vi "CAN BL Node Check.vi"(5 "TimeOut":u32, 6 "pType":u32, 7 "pVersion":u32, 9 "NodeAddr":u16, 10 "CANIndex":i32, 11 "DevHandle":i32) -> (2 "function return":i32, 3 "pVersion out":u32, 4 "pType out":u32)   [LabVIEW 2010, in "usb2can.lvlib"]
doc: "int WINAPI CAN_BL_NodeCheck(int DevHandle,int CANIndex,unsigned short NodeAddr,unsigned int *pVersion,unsigned int *pType,unsigned int TimeOut);"
uses:
  usb2can.lvlib
  USB2XXX.dll
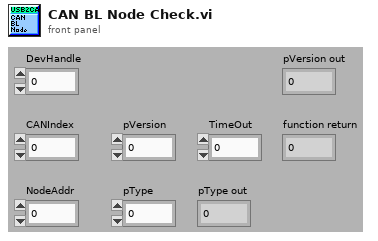
[diagram p1: front panel]
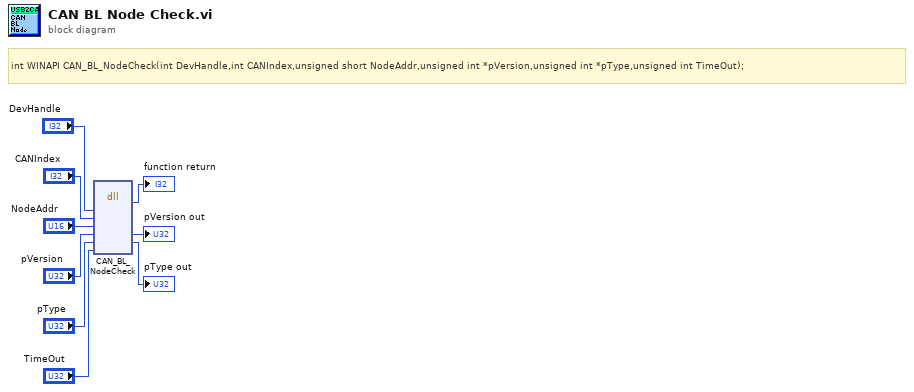
[diagram p0: block diagram]
diagram:
  # "int WINAPI CAN_BL_NodeCheck(int DevHandle,int CANIndex,unsigned short NodeAddr,unsigned int *pVersion,unsigned int *pType,unsigned int TimeOut);"
  n1 = dll-call lib="G:/OtherWork/USB2XXX_Example/trunk/Labview/PublicFiles/usb2can/USB2XXX.*" fn="CAN_BL_NodeCheck"("DevHandle"="DevHandle", "CANIndex"="CANIndex", "NodeAddr"="NodeAddr", "pVersion"="pVersion", "pType"="pType", "TimeOut"="TimeOut") -> (→"function return":i32, "pVersion"=→"pVersion out":u32, "pType"=→"pType out":u32)  [unwired: 7 in, 2 out]
